vi "ParseResponse-test.vi"(7 "datatype":i32[](array[numeric]), 8 "error in (no error)":errorcluster, 10 "{JSON}":string) -> (0 "error out":errorcluster, 1 "id":string, 2 "data out":i32[](array[numeric]), 4 "reversed":string)   [LabVIEW 2019]
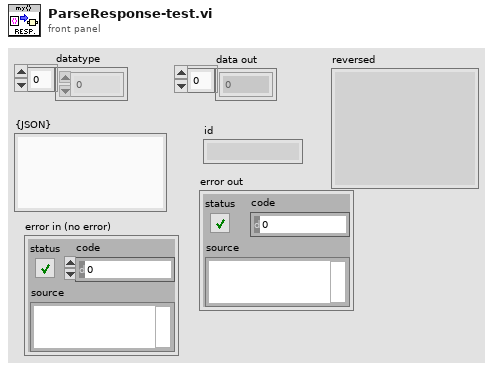
[diagram p1: front panel]
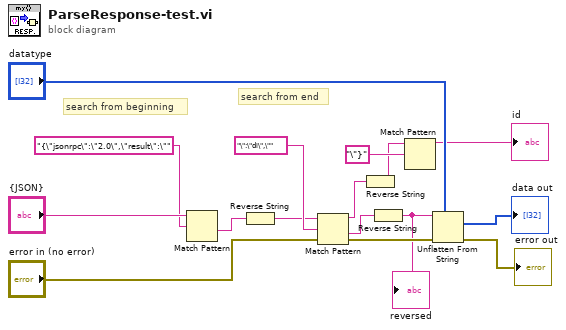
[diagram p0: block diagram]
diagram:
  # "search from end"
  # "search from beginning"
  n1 = Match Pattern(string="{JSON}", regular expression="{\"jsonrpc\":\"2.0\",\"result\":\"") -> (after substring=w2:string)  [unwired: 1 in, 3 out]
  n2 = Reverse String(1:w2) -> (0:w3:string)
  n3 = Match Pattern(string=w3, regular expression="\":\"di\",\"") -> (before substring=w9:string, after substring=w5:string)  [unwired: 1 in, 2 out]
  n4 = Reverse String(1:w9) -> (0:w10:string)
  n5 = Reverse String(1:w5) -> (0:w6:string)
  "reversed" <- w6
  n6 = Match Pattern(string=w10, regular expression="\"}") -> (before substring=→"id":string)  [unwired: 1 in, 3 out]
  n7 = Unflatten From String(type="datatype", binary string=w6, error in (no error)="error in (no error)") -> (value=→"data out":i32[], error out=→"error out":errorcluster)  [unwired: 2 in, 1 out]
